vi "配置文件-以数组形式输出.vi"(4 "默认值":string[](array[string]), 6 "create file if necessary (T)":bool=TRUE, 8 "error in (no error)":errorcluster caption="错误输入（无错误）", 9 "键名":string[](array[string]), 10 "章名":string[](array[string]), 11 "路径":string) -> (0 "error out":errorcluster caption="错误输出", 3 "输出值":string[][](array[string]))   [LabVIEW 2014]
doc: "该模板用于创建子VI。"
uses:
  <vilib>/Utility/config.llb/NI_LVConfig.lvlib
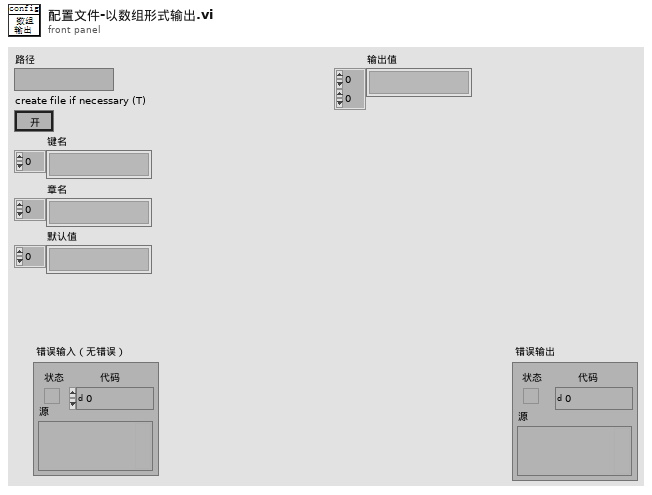
[diagram p1: front panel]
types:
  T1 = typedef "NI_LVConfig.lvlib/Config Data RefNum.ctl" = refnum<k1>
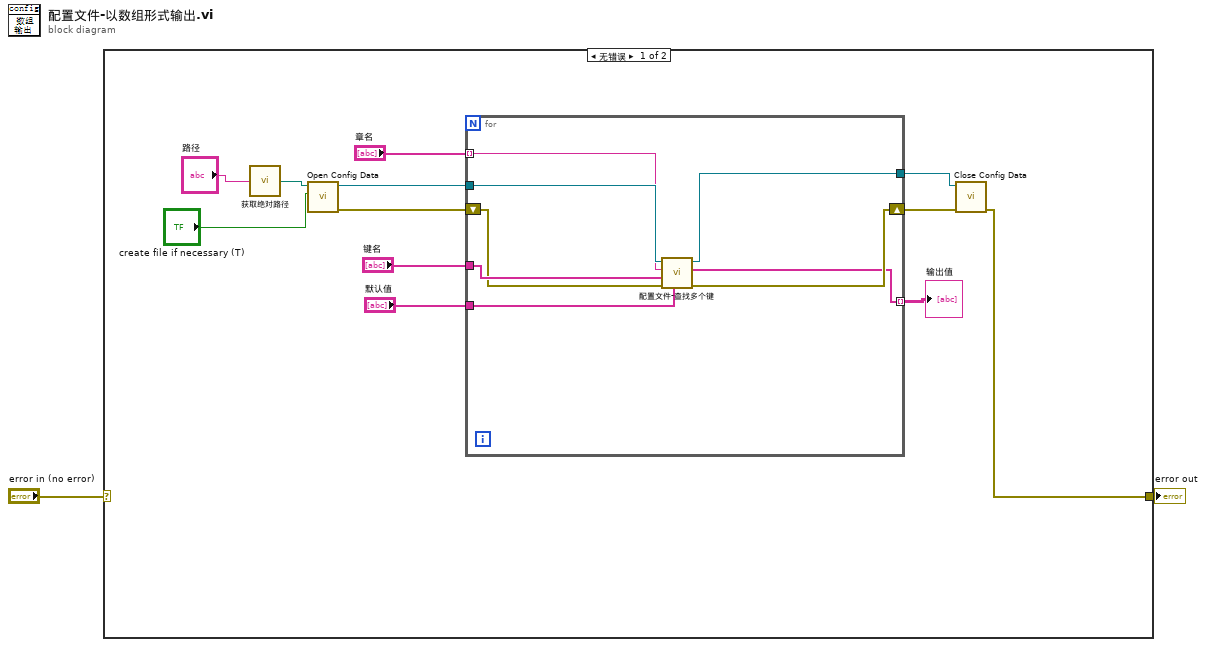
[diagram p0: block diagram]
diagram:
  n1 = case shown="无错误" "error in (no error)" {
    selector: "error in (no error)" -> [_ w23]
    tunnel: [w4 w23] -> w1
    frame No Error {
      n2 = call "获取绝对路径.vi"("relativePath"="路径") -> ("absolutePath"=w13:path)
      n3 = call <vilib>:"Open Config Data.vi"("create file if necessary (T)"="create file if necessary (T)", "configuration file path"=w13) -> ("error out"=w10:errorcluster, "refnum"=w11:T1)  [unwired: 7 in, 1 out]
      n4 = for {
        tunnel: w11 -> [w21]
        shift-right: [w18] -> w5
        shift-left: w10 -> [w19]
        tunnel: "章名" -> [w20] mode=indexing
        tunnel: "键名" -> [w22]
        tunnel: "默认值" -> [w15]
        tunnel: [w17] -> w6
        tunnel: [w16] -> w3 mode=indexing
        n5 = call "配置文件-查找多个键.vi"("默认值"=w15, "错误输入（无错误）"=w19, "键名"=w22, "章名"=w20, "引用句柄输入"=w21) -> ("错误输出"=w18:errorcluster, "查询结果"=w16:string[], "引用句柄输出"=w17:T1)  [unwired: 4 in]
      }
      "输出值" <- w3
      n6 = call <vilib>:"Close Config Data.vi"("error in (no error)"=w5, "refnum"=w6) -> ("error out"=w4:errorcluster)  [unwired: 8 in, 1 out]
    }
    frame Error {
    }
  }
  "error out" <- w1
